vi "TargetVI.vi"(9 "Wait (ms)":u32=1000, 10 "Y":dbl, 11 "X":dbl) -> (3 "X + Y":dbl)   [LabVIEW 2021]
doc: "Target VI used in conjunction with the asynchronous call examples."
panel:
  out "Elapsed Time (s)":dbl format="%.1g"
  # "Target VI used with the asynchronous call examples."
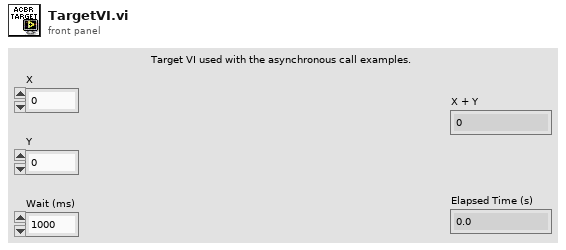
[diagram p1: front panel]
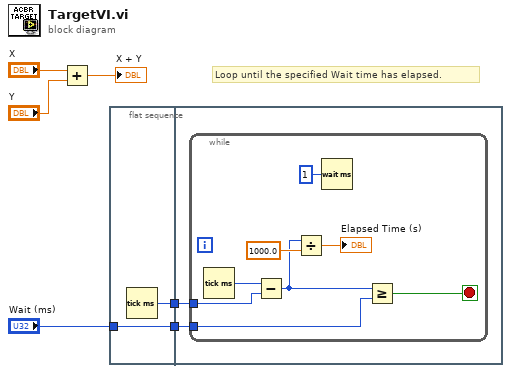
[diagram p0: block diagram]
diagram:
  # "Loop until the specified Wait time has elapsed."
  n1 = Add(x="X", y="Y") -> (x+y=→"X + Y":dbl)
  n2 = flat-sequence {
    tunnel: [w8] -> w3
    tunnel: [w7] -> w2
    tunnel: "Wait (ms)" -> [w7]
    tunnel: w3 -> [w10]
    tunnel: w2 -> [w9]
    frame #0 {
      n3 = Tick Count (ms)() -> (millisecond timer value=w8:u32)
    }
    frame #1 {
      n4 = while {
        tunnel: w10 -> [w16]
        tunnel: w9 -> [w14]
        stop <- w15 stop-if-true
        n5 = Tick Count (ms)() -> (millisecond timer value=w13:u32)
        n6 = Subtract(x=w13, y=w16) -> (x-y=w12:u32)
        n7 = Divide(x=w12, y=1000.0) -> (x/y=→"Elapsed Time (s)":dbl)
        n8 = Wait (ms)(milliseconds to wait=u32 1) -> ()  [unwired: 1 out]
        n9 = Greater Or Equal?(x=w12, y=w14) -> (x >= y?=w15:bool)
      }
    }
  }
